vi "IMU Get Quaternion.vi"(8 "error in (no error)":errorcluster) -> (0 "error out":errorcluster, 2 "timestamp":i64, 3 "quaternion":T1)   [LabVIEW 2026, in "MrcLib.lvlib"]
doc: "Return the bearing of the robot controller in a Quaternion."
uses:
  MrcLib.lvlib
  Types/MRC Quaternion Values.ctl
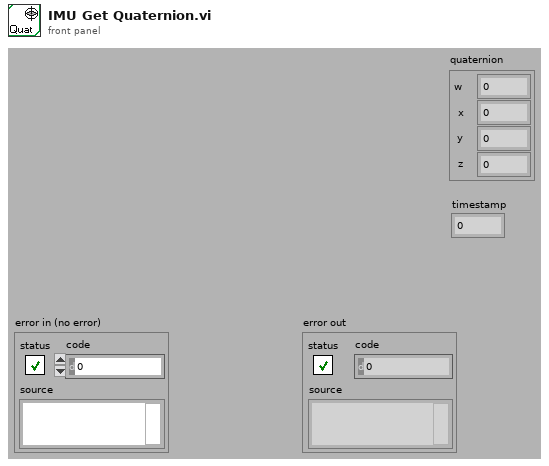
[diagram p1: front panel]
types:
  T1 = typedef "MrcLib.lvlib/MRC Quaternion Values.ctl" = cluster{"w":dbl, "x":dbl, "y":dbl, "z":dbl}
  T2 = typedef "MrcLib.lvlib/MRC Quaternion.ctl" = cluster{"timestamp":i64, "w":dbl, "x":dbl, "y":dbl, "z":dbl}
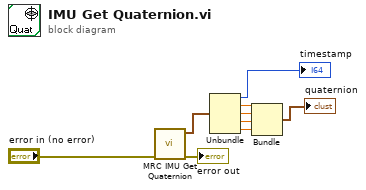
[diagram p0: block diagram]
diagram:
  n1 = call "MRC IMU Get Quaternion.vi"("error in (no error)"="error in (no error)") -> ("error out"=→"error out":errorcluster, "quaternion out"=w7:T2)  [unwired: 9 in]
  n2 = Unbundle(w7) -> ("timestamp"=→"timestamp":i64, "w"=w6:dbl, "x"=w5:dbl, "y"=w4:dbl, "z"=w3:dbl)
  n3 = Bundle("w"=w6, "x"=w5, "y"=w4, "z"=w3) -> (→"quaternion":cluster{"w":dbl, "x":dbl, "y":dbl, "z":dbl})  [unwired: 1 in]
